vi "fakePatternedImage.vi"(10 "current location":T2, 11 "read output":T1) -> (3 "read output out":T1)   [LabVIEW 2010]
uses:
  common_typedefs/channels_cluster.ctl
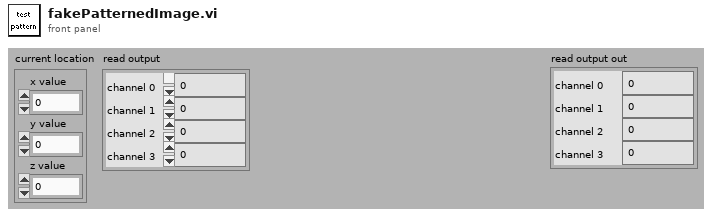
[diagram p1: front panel]
types:
  T1 = typedef "channels_cluster.ctl" = cluster{"channel 0":u32, "channel 1":u32, "channel 2":u32, "channel 3":u32}
  T2 = cluster{"x value":i16, "y value":i16, "z value":i16}
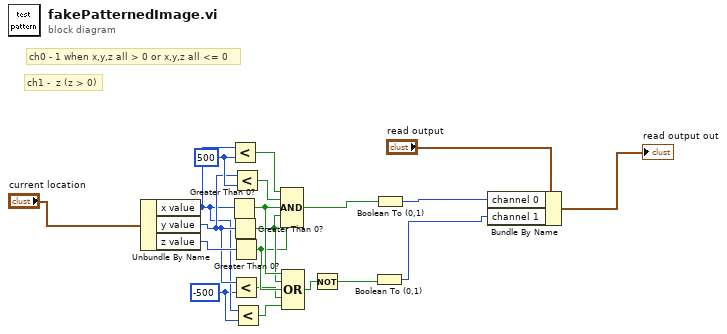
[diagram p0: block diagram]
diagram:
  w3 = i16 -500 ("y")
  w8 = i16 500 ("y")
  # "ch1 -  z (z > 0)"
  # "ch0 - 1 when x,y,z all > 0 or x,y,z all <= 0"
  n1 = Unbundle By Name("current location") -> ("x value"=w4:i16, "y value"=w5:i16, "z value"=w13:i16)
  n2 = Greater Than 0?(x=w4) -> (x > 0?=w19:bool)
  n3 = Less?(x=w4, y=w8) -> (x < y?=w7:bool)
  n4 = Greater Than 0?(x=w5) -> (x > 0?=w18:bool)
  n5 = Greater Than 0?(x=w13) -> (x > 0?=w12:bool)
  n6 = Less?(x=w5, y=w3) -> (x < y?=w1:bool)
  n7 = Less?(x=w5, y=w8) -> (x < y?=w6:bool)
  n8 = Less?(x=w4, y=w3) -> (x < y?=w2:bool)
  n9 = Compound Arithmetic op=AND(w7, w6, w19, w18, w12) -> (w11:bool)
  n10 = Compound Arithmetic op=OR(w19, w18, w12, w1, w2) -> (w17:bool)
  n11 = Not(x=w17) -> (.not. x?=w10:bool)
  n12 = Boolean To (0,1)(Boolean=w10) -> (0, 1=w9:i16)
  n13 = Boolean To (0,1)(Boolean=w11) -> (0, 1=w14:i16)
  n14 = Bundle By Name(cluster="read output", "channel 0"=w14, "channel 1"=w9) -> (→"read output out":T1)
